vi "Methods to Method Info.vi"(10 "Class":string, 11 "Methods from Node":T2(array[cluster])) -> (2 "Methods for Tree":T1(array[cluster]), 3 "Methods[]":T3(array[cluster])=[{"Class Info"={"Unique ID string"="1", "Parent ID string"="", "Class Name (unlocalized)"="Application", "Class Name (localized)"="Application"}, "Method Info"={"Unique ID string"="7d0", "Data name"="Print.Function To Printer", "Short name (localized)"="Print.Function To Printer", "Long name (localized)"="Print:Function To Printer"}, "Method Flags"={"IsDeprecated"=FALSE, "IsPrivate"=TRUE, "IsScripting"=FALSE, "IsNotInRun-Time"=TRUE}, "Divider"=FALSE}, {"Class Info"={"Unique ID string"="1", "Parent ID string"="", "Class Name (unlocalized)"="Application", "Class Name (localized)"="Application"}, "Method Info"={"Unique ID string"="7d5", "Data name"="Mass Compile", "Short name (localized)"="Mass Compile", "Long name (localized)"="Mass Compile"}, "Method Flags"={"IsDeprecated"=FALSE, "IsPrivate"=FALSE, "IsScripting"=FALSE, "IsNotInRun-Time"=TRUE}, "Divider"=FALSE}, {"Class Info"={"Unique ID string"="1", "Parent ID string"="", "Class Name (unlocalized)"="Application", "Class Name (localized)"="Application"}, "Method Info"={"Unique ID string"="7d6", "Data name"="UI.Cmp VIs", "Short name (localized)"="UI.Cmp VIs", "Long name (localized)"="User Interaction:Compare VIs"}, "Method Flags"={"IsDeprecated"=FALSE, "IsPrivate"=TRUE, "IsScripting"=FALSE, "IsNotInRun-Time"=TRUE}, "Divider"=FALSE}, {"Class Info"={"Unique ID string"="1", "Parent ID string"="", "Class Name (unlocalized)"="Application", "Class Name (localized)"="Application"}, "Method Info"={"Unique ID string"="7da", "Data name"="History Since", "Short name (localized)"="History Since", "Long name (localized)"="History Since"}, "Method Flags"={"IsDeprecated"=FALSE, "IsPrivate"=TRUE, "IsScripting"=FALSE, "IsNotInRun-Time"=TRUE}, "Divider"=FALSE}, {"Class Info"={"Unique ID string"="1", "Parent ID string"="", "Class Name (unlocalized)"="Application", "Class Name (localized)"="Application"}, "Method Info"={"Unique ID string"="7de", "Data name"="Bring To Front", "Short name (localized)"="Bring To Front", "Long name (localized)"="Bring To Front"}, "Method Flags"={"IsDeprecated"=FALSE, "IsPrivate"=FALSE, "IsScripting"=FALSE, "IsNotInRun-Time"=FALSE}, "Divider"=FALSE}, {"Class Info"={"Unique ID string"="1", "Parent ID string"="", "Class Name (unlocalized)"="Application", "Class Name (localized)"="Application"}, "Method Info"={"Unique ID string"="7e0", "Data name"="Build.Application", "Short name (localized)"="Build.Application", "Long name (localized)"="Build:Application"}, "Method Flags"={"IsDeprecated"=FALSE, "IsPrivate"=TRUE, "IsScripting"=FALSE, "IsNotInRun-Time"=TRUE}, "Divider"=FALSE}, {"Class Info"={"Unique ID string"="1", "Parent ID string"="", "Class Name (unlocalized)"="Application", "Class Name (localized)"="Application"}, "Method Info"={"Unique ID string"="7e1", "Data name"="Build.Distribution", "Short name (localized)"="Build.Distribution", "Long name (localized)"="Build:Distribution"}, "Method Flags"={"IsDeprecated"=FALSE, "IsPrivate"=TRUE, "IsScripting"=FALSE, "IsNotInRun-Time"=TRUE}, "Divider"=FALSE}, {"Class Info"={"Unique ID string"="1", "Parent ID string"="", "Class Name (unlocalized)"="Application", "Class Name (localized)"="Application"}, "Method Info"={"Unique ID string"="7e3", "Data name"="Disconnect From Slave", "Short name (localized)"="Disconnect From Slave", "Long name (localized)"="LVRT:Disconnect From Slave"}, "Method Flags"={"IsDeprecated"=FALSE, "IsPrivate"=FALSE, "IsScripting"=FALSE, "IsNotInRun-Time"=TRUE}, "Divider"=FALSE}, {"Class Info"={"Unique ID string"="1", "Parent ID string"="", "Class Name (unlocalized)"="Application", "Class Name (localized)"="Application"}, "Method Info"={"Unique ID string"="7e4", "Data name"="LVRT.Check DLLs", "Short name (localized)"="LVRT.Check DLLs", "Long name (localized)"="LVRT:Check DLLs"}, "Method Flags"={"IsDeprecated"=FALSE, "IsPrivate"=TRUE, "IsScripting"=FALSE, "IsNotInRun-Time"=TRUE}, "Divider"=FALSE}, {"Class Info"={"Unique ID string"="1", "Parent ID string"="", "Class Name (unlocalized)"="Application", "Class Name (localized)"="Application"}, "Method Info"={"Unique ID string"="7e6", "Data name"="Call Internal Cmd", "Short name (localized)"="Call Internal Cmd", "Long name (localized)"="Call Internal Command"}, "Method Flags"={"IsDeprecated"=FALSE, "IsPrivate"=TRUE, "IsScripting"=FALSE, "IsNotInRun-Time"=FALSE}, "Divider"=FALSE}, {"Class Info"={"Unique ID string"="1", "Parent ID string"="", "Class Name (unlocalized)"="Application", "Class Name (localized)"="Application"}, "Method Info"={"Unique ID string"="7e7", "Data name"="Query Internal Operation Tracking Data", "Short name (localized)"="Query Internal Operation Tracking Data", "Long name (localized)"="Query Internal Operation Tracking Data"}, "Method Flags"={"IsDeprecated"=FALSE, "IsPrivate"=TRUE, "IsScripting"=FALSE, "IsNotInRun-Time"=FALSE}, "Divider"=FALSE}, {"Class Info"={"Unique ID string"="1", "Parent ID string"="", "Class Name (unlocalized)"="Application", "Class Name (localized)"="Application"}, "Method Info"={"Unique ID string"="7e8", "Data name"="Class Operator.Get", "Short name (localized)"="Class Operator.Get", "Long name (localized)"="Class Operator:Get"}, "Method Flags"={"IsDeprecated"=FALSE, "IsPrivate"=FALSE, "IsScripting"=TRUE, "IsNotInRun-Time"=FALSE}, "Divider"=FALSE}, {"Class Info"={"Unique ID string"="1", "Parent ID string"="", "Class Name (unlocalized)"="Application", "Class Name (localized)"="Application"}, "Method Info"={"Unique ID string"="7e9", "Data name"="Class Operator.Set", "Short name (localized)"="Class Operator.Set", "Long name (localized)"="Class Operator:Set"}, "Method Flags"={"IsDeprecated"=FALSE, "IsPrivate"=FALSE, "IsScripting"=TRUE, "IsNotInRun-Time"=FALSE}, "Divider"=FALSE}, {"Class Info"={"Unique ID string"="1", "Parent ID string"="", "Class Name (unlocalized)"="Application", "Class Name (localized)"="Application"}, "Method Info"={"Unique ID string"="7ea", "Data name"="Class Operator.Remove", "Short name (localized)"="Class Operator.Remove", "Long name (localized)"="Class Operator:Remove"}, "Method Flags"={"IsDeprecated"=FALSE, "IsPrivate"=FALSE, "IsScripting"=TRUE, "IsNotInRun-Time"=FALSE}, "Divider"=FALSE}, {"Class Info"={"Unique ID string"="1", "Parent ID string"="", "Class Name (unlocalized)"="Application", "Class Name (localized)"="Application"}, "Method Info"={"Unique ID string"="7eb", "Data name"="Class Operator.Remove All", "Short name (localized)"="Class Operator.Remove All", "Long name (localized)"="Class Operator:Remove All"}, "Method Flags"={"IsDeprecated"=FALSE, "IsPrivate"=FALSE, "IsScripting"=TRUE, "IsNotInRun-Time"=FALSE}, "Divider"=FALSE}, {"Class Info"={"Unique ID string"="1", "Parent ID string"="", "Class Name (unlocalized)"="Application", "Class Name (localized)"="Application"}, "Method Info"={"Unique ID string"="7ed", "Data name"="Clipboard.Get Image", "Short name (localized)"="Clipboard.Get Image", "Long name (localized)"="Clipboard:Get Image"}, "Method Flags"={"IsDeprecated"=FALSE, "IsPrivate"=FALSE, "IsScripting"=FALSE, "IsNotInRun-Time"=FALSE}, "Divider"=FALSE}, {"Class Info"={"Unique ID string"="1", "Parent ID string"="", "Class Name (unlocalized)"="Application", "Class Name (localized)"="Application"}, "Method Info"={"Unique ID string"="7ee", "Data name"="RP.Server Network Load", "Short name (localized)"="RP.Server Network Load", "Long name (localized)"="Remote Panel:Server Network Load"}, "Method Flags"={"IsDeprecated"=FALSE, "IsPrivate"=TRUE, "IsScripting"=FALSE, "IsNotInRun-Time"=FALSE}, "Divider"=FALSE}, {"Class Info"={"Unique ID string"="1", "Parent ID string"="", "Class Name (unlocalized)"="Application", "Class Name (localized)"="Application"}, "Method Info"={"Unique ID string"="7ef", "Data name"="Clipboard.Empty", "Short name (localized)"="Clipboard.Empty", "Long name (localized)"="Clipboard:Empty"}, "Method Flags"={"IsDeprecated"=FALSE, "IsPrivate"=FALSE, "IsScripting"=TRUE, "IsNotInRun-Time"=TRUE}, "Divider"=FALSE}, {"Class Info"={"Unique ID string"="1", "Parent ID string"="", "Class Name (unlocalized)"="Application", "Class Name (localized)"="Application"}, "Method Info"={"Unique ID string"="7f1", "Data name"="RP.Open Connection To Server", "Short name (localized)"="RP.Open Connection To Server", "Long name (localized)"="Remote Panel:Open Connection To Server"}, "Method Flags"={"IsDeprecated"=FALSE, "IsPrivate"=FALSE, "IsScripting"=FALSE, "IsNotInRun-Time"=FALSE}, "Divider"=FALSE}, {"Class Info"={"Unique ID string"="1", "Parent ID string"="", "Class Name (unlocalized)"="Application", "Class Name (localized)"="Application"}, "Method Info"={"Unique ID string"="7f2", "Data name"="RP.Client Network Load", "Short name (localized)"="RP.Client Network Load", "Long name (localized)"="Remote Panel:Client Network Load"}, "Method Flags"={"IsDeprecated"=FALSE, "IsPrivate"=TRUE, "IsScripting"=FALSE, "IsNotInRun-Time"=FALSE}, "Divider"=FALSE}, {"Class Info"={"Unique ID string"="1", "Parent ID string"="", "Class Name (unlocalized)"="Application", "Class Name (localized)"="Application"}, "Method Info"={"Unique ID string"="7f3", "Data name"="Compile VIs Needing Compilation", "Short name (localized)"="Compile VIs Needing Compilation", "Long name (localized)"="Compile VIs Needing Compilation"}, "Method Flags"={"IsDeprecated"=FALSE, "IsPrivate"=TRUE, "IsScripting"=FALSE, "IsNotInRun-Time"=TRUE}, "Divider"=FALSE}, {"Class Info"={"Unique ID string"="1", "Parent ID string"="", "Class Name (unlocalized)"="Application", "Class Name (localized)"="Application"}, "Method Info"={"Unique ID string"="7f4", "Data name"="UI.Show Inplaceness Terminals", "Short name (localized)"="UI.Show Inplaceness Terminals", "Long name (localized)"="User Interaction:Show Inplaceness Terminals"}, "Method Flags"={"IsDeprecated"=FALSE, "IsPrivate"=TRUE, "IsScripting"=FALSE, "IsNotInRun-Time"=TRUE}, "Divider"=FALSE}, {"Class Info"={"Unique ID string"="1", "Parent ID string"="", "Class Name (unlocalized)"="Application", "Class Name (localized)"="Application"}, "Method Info"={"Unique ID string"="7f7", "Data name"="Conn Responsive.Check", "Short name (localized)"="Conn Responsive.Check", "Long name (localized)"="Connection Responsiveness:Check"}, "Method Flags"={"IsDeprecated"=FALSE, "IsPrivate"=FALSE, "IsScripting"=FALSE, "IsNotInRun-Time"=FALSE}, "Divider"=FALSE}, {"Class Info"={"Unique ID string"="1", "Parent ID string"="", "Class Name (unlocalized)"="Application", "Class Name (localized)"="Application"}, "Method Info"={"Unique ID string"="7f8", "Data name"="Conn Responsive.Info", "Short name (localized)"="Conn Responsive.Info", "Long name (localized)"="Connection Responsiveness:Information"}, "Method Flags"={"IsDeprecated"=FALSE, "IsPrivate"=FALSE, "IsScripting"=FALSE, "IsNotInRun-Time"=FALSE}, "Divider"=FALSE}, {"Class Info"={"Unique ID string"="1", "Parent ID string"="", "Class Name (unlocalized)"="Application", "Class Name (localized)"="Application"}, "Method Info"={"Unique ID string"="7f9", "Data name"="Get VI Version", "Short name (localized)"="Get VI Version", "Long name (localized)"="Get VI:Version"}, "Method Flags"={"IsDeprecated"=FALSE, "IsPrivate"=FALSE, "IsScripting"=FALSE, "IsNotInRun-Time"=FALSE}, "Divider"=FALSE}, {"Class Info"={"Unique ID string"="1", "Parent ID string"="", "Class Name (unlocalized)"="Application", "Class Name (localized)"="Application"}, "Method Info"={"Unique ID string"="7fa", "Data name"="UI.PlacePaletteObjOnCursor", "Short name (localized)"="UI.PlacePaletteObjOnCursor", "Long name (localized)"="User Interaction:Place Palette Object on Cursor"}, "Method Flags"={"IsDeprecated"=FALSE, "IsPrivate"=FALSE, "IsScripting"=TRUE, "IsNotInRun-Time"=TRUE}, "Divider"=FALSE}, {"Class Info"={"Unique ID string"="1", "Parent ID string"="", "Class Name (unlocalized)"="Application", "Class Name (localized)"="Application"}, "Method Info"={"Unique ID string"="7fb", "Data name"="Browse DataSocket", "Short name (localized)"="Browse DataSocket", "Long name (localized)"="Browse DataSocket"}, "Method Flags"={"IsDeprecated"=FALSE, "IsPrivate"=FALSE, "IsScripting"=FALSE, "IsNotInRun-Time"=FALSE}, "Divider"=FALSE}, {"Class Info"={"Unique ID string"="1", "Parent ID string"="", "Class Name (unlocalized)"="Application", "Class Name (localized)"="Application"}, "Method Info"={"Unique ID string"="7fd", "Data name"="UI.Hilight Pal Menu Item", "Short name (localized)"="UI.Hilight Pal Menu Item", "Long name (localized)"="User Interaction:Hilight Palette Menu Item"}, "Method Flags"={"IsDeprecated"=FALSE, "IsPrivate"=FALSE, "IsScripting"=TRUE, "IsNotInRun-Time"=TRUE}, "Divider"=FALSE}, {"Class Info"={"Unique ID string"="1", "Parent ID string"="", "Class Name (unlocalized)"="Application", "Class Name (localized)"="Application"}, "Method Info"={"Unique ID string"="7ff", "Data name"="New LabVIEW Document", "Short name (localized)"="New LabVIEW Document", "Long name (localized)"="New LabVIEW Document"}, "Method Flags"={"IsDeprecated"=FALSE, "IsPrivate"=FALSE, "IsScripting"=TRUE, "IsNotInRun-Time"=TRUE}, "Divider"=FALSE}, {"Class Info"={"Unique ID string"="1", "Parent ID string"="", "Class Name (unlocalized)"="Application", "Class Name (localized)"="Application"}, "Method Info"={"Unique ID string"="800", "Data name"="Pwd.Clear Cache", "Short name (localized)"="Pwd.Clear Cache", "Long name (localized)"="Password:Clear Cache"}, "Method Flags"={"IsDeprecated"=FALSE, "IsPrivate"=TRUE, "IsScripting"=FALSE, "IsNotInRun-Time"=FALSE}, "Divider"=FALSE}, {"Class Info"={"Unique ID string"="1", "Parent ID string"="", "Class Name (unlocalized)"="Application", "Class Name (localized)"="Application"}, "Method Info"={"Unique ID string"="801", "Data name"="Pwd.Add To Cache", "Short name (localized)"="Pwd.Add To Cache", "Long name (localized)"="Password:Add To Cache"}, "Method Flags"={"IsDeprecated"=FALSE, "IsPrivate"=TRUE, "IsScripting"=FALSE, "IsNotInRun-Time"=FALSE}, "Divider"=FALSE}, {"Class Info"={"Unique ID string"="1", "Parent ID string"="", "Class Name (unlocalized)"="Application", "Class Name (localized)"="Application"}, "Method Info"={"Unique ID string"="802", "Data name"="RP.Close Connection To Server", "Short name (localized)"="RP.Close Connection To Server", "Long name (localized)"="Remote Panel:Close Connection To Server"}, "Method Flags"={"IsDeprecated"=FALSE, "IsPrivate"=FALSE, "IsScripting"=FALSE, "IsNotInRun-Time"=FALSE}, "Divider"=FALSE}, {"Class Info"={"Unique ID string"="1", "Parent ID string"="", "Class Name (unlocalized)"="Application", "Class Name (localized)"="Application"}, "Method Info"={"Unique ID string"="803", "Data name"="RP.Client Request Control", "Short name (localized)"="RP.Client Request Control", "Long name (localized)"="Remote Panel:Client Request Control"}, "Method Flags"={"IsDeprecated"=FALSE, "IsPrivate"=FALSE, "IsScripting"=FALSE, "IsNotInRun-Time"=FALSE}, "Divider"=FALSE}, {"Class Info"={"Unique ID string"="1", "Parent ID string"="", "Class Name (unlocalized)"="Application", "Class Name (localized)"="Application"}, "Method Info"={"Unique ID string"="804", "Data name"="RP.Client Release Control", "Short name (localized)"="RP.Client Release Control", "Long name (localized)"="Remote Panel:Client Release Control"}, "Method Flags"={"IsDeprecated"=FALSE, "IsPrivate"=FALSE, "IsScripting"=FALSE, "IsNotInRun-Time"=FALSE}, "Divider"=FALSE}, {"Class Info"={"Unique ID string"="1", "Parent ID string"="", "Class Name (unlocalized)"="Application", "Class Name (localized)"="Application"}, "Method Info"={"Unique ID string"="805", "Data name"="Get VI.Title", "Short name (localized)"="Get VI.Title", "Long name (localized)"="Get VI:Title"}, "Method Flags"={"IsDeprecated"=FALSE, "IsPrivate"=FALSE, "IsScripting"=FALSE, "IsNotInRun-Time"=FALSE}, "Divider"=FALSE}, {"Class Info"={"Unique ID string"="1", "Parent ID string"="", "Class Name (unlocalized)"="Application", "Class Name (localized)"="Application"}, "Method Info"={"Unique ID string"="806", "Data name"="Get VI.Description", "Short name (localized)"="Get VI.Description", "Long name (localized)"="Get VI:Description"}, "Method Flags"={"IsDeprecated"=FALSE, "IsPrivate"=FALSE, "IsScripting"=FALSE, "IsNotInRun-Time"=FALSE}, "Divider"=FALSE}, {"Class Info"={"Unique ID string"="1", "Parent ID string"="", "Class Name (unlocalized)"="Application", "Class Name (localized)"="Application"}, "Method Info"={"Unique ID string"="807", "Data name"="Add Probe To Cache", "Short name (localized)"="Add Probe To Cache", "Long name (localized)"="Add Probe To Cache"}, "Method Flags"={"IsDeprecated"=FALSE, "IsPrivate"=TRUE, "IsScripting"=FALSE, "IsNotInRun-Time"=FALSE}, "Divider"=FALSE}, {"Class Info"={"Unique ID string"="1", "Parent ID string"="", "Class Name (unlocalized)"="Application", "Class Name (localized)"="Application"}, "Method Info"={"Unique ID string"="809", "Data name"="Create COM WDT Data", "Short name (localized)"="Create COM WDT Data", "Long name (localized)"="Create COM WDT Data"}, "Method Flags"={"IsDeprecated"=FALSE, "IsPrivate"=TRUE, "IsScripting"=FALSE, "IsNotInRun-Time"=FALSE}, "Divider"=FALSE}, {"Class Info"={"Unique ID string"="1", "Parent ID string"="", "Class Name (unlocalized)"="Application", "Class Name (localized)"="Application"}, "Method Info"={"Unique ID string"="80a", "Data name"="Image Data To Byte Array", "Short name (localized)"="Image Data To Byte Array", "Long name (localized)"="Image Data To Byte Array"}, "Method Flags"={"IsDeprecated"=FALSE, "IsPrivate"=TRUE, "IsScripting"=FALSE, "IsNotInRun-Time"=FALSE}, "Divider"=FALSE}, {"Class Info"={"Unique ID string"="1", "Parent ID string"="", "Class Name (unlocalized)"="Application", "Class Name (localized)"="Application"}, "Method Info"={"Unique ID string"="80b", "Data name"=".NET.Get Assembly Full Name", "Short name (localized)"=".NET.Get Assembly Full Name", "Long name (localized)"=".NET:Get Assembly Full Name"}, "Method Flags"={"IsDeprecated"=FALSE, "IsPrivate"=TRUE, "IsScripting"=FALSE, "IsNotInRun-Time"=TRUE}, "Divider"=FALSE}, {"Class Info"={"Unique ID string"="1", "Parent ID string"="", "Class Name (unlocalized)"="Application", "Class Name (localized)"="Application"}, "Method Info"={"Unique ID string"="80c", "Data name"=".NET.Convert To .NET Type", "Short name (localized)"=".NET.Convert To .NET Type", "Long name (localized)"=".NET:Convert To .NET Type"}, "Method Flags"={"IsDeprecated"=FALSE, "IsPrivate"=TRUE, "IsScripting"=FALSE, "IsNotInRun-Time"=FALSE}, "Divider"=FALSE}, {"Class Info"={"Unique ID string"="1", "Parent ID string"="", "Class Name (unlocalized)"="Application", "Class Name (localized)"="Application"}, "Method Info"={"Unique ID string"="80d", "Data name"=".NET.Convert Obj To LV Variant", "Short name (localized)"=".NET.Convert Obj To LV Variant", "Long name (localized)"=".NET:Convert Object To LabVIEW Variant"}, "Method Flags"={"IsDeprecated"=FALSE, "IsPrivate"=TRUE, "IsScripting"=FALSE, "IsNotInRun-Time"=FALSE}, "Divider"=FALSE}, {"Class Info"={"Unique ID string"="1", "Parent ID string"="", "Class Name (unlocalized)"="Application", "Class Name (localized)"="Application"}, "Method Info"={"Unique ID string"="80e", "Data name"="Get Pal Menu Info", "Short name (localized)"="Get Pal Menu Info", "Long name (localized)"="Palettes:Get Menu Information"}, "Method Flags"={"IsDeprecated"=FALSE, "IsPrivate"=TRUE, "IsScripting"=FALSE, "IsNotInRun-Time"=TRUE}, "Divider"=FALSE}, {"Class Info"={"Unique ID string"="1", "Parent ID string"="", "Class Name (unlocalized)"="Application", "Class Name (localized)"="Application"}, "Method Info"={"Unique ID string"="810", "Data name"="C TypeDefs.Reset", "Short name (localized)"="C TypeDefs.Reset", "Long name (localized)"="C TypeDefs:Reset"}, "Method Flags"={"IsDeprecated"=FALSE, "IsPrivate"=TRUE, "IsScripting"=FALSE, "IsNotInRun-Time"=FALSE}, "Divider"=FALSE}, {"Class Info"={"Unique ID string"="1", "Parent ID string"="", "Class Name (unlocalized)"="Application", "Class Name (localized)"="Application"}, "Method Info"={"Unique ID string"="811", "Data name"="C TypeDefs.Get", "Short name (localized)"="C TypeDefs.Get", "Long name (localized)"="C TypeDefs:Get"}, "Method Flags"={"IsDeprecated"=FALSE, "IsPrivate"=TRUE, "IsScripting"=FALSE, "IsNotInRun-Time"=FALSE}, "Divider"=FALSE}, {"Class Info"={"Unique ID string"="1", "Parent ID string"="", "Class Name (unlocalized)"="Application", "Class Name (localized)"="Application"}, "Method Info"={"Unique ID string"="812", "Data name"="Context.OpenSibling", "Short name (localized)"="Context.OpenSibling", "Long name (localized)"="Context:Open Sibling"}, "Method Flags"={"IsDeprecated"=FALSE, "IsPrivate"=TRUE, "IsScripting"=FALSE, "IsNotInRun-Time"=FALSE}, "Divider"=FALSE}, {"Class Info"={"Unique ID string"="1", "Parent ID string"="", "Class Name (unlocalized)"="Application", "Class Name (localized)"="Application"}, "Method Info"={"Unique ID string"="813", "Data name"="Project.Open", "Short name (localized)"="Project.Open", "Long name (localized)"="Project:Open"}, "Method Flags"={"IsDeprecated"=FALSE, "IsPrivate"=FALSE, "IsScripting"=FALSE, "IsNotInRun-Time"=FALSE}, "Divider"=FALSE}, {"Class Info"={"Unique ID string"="1", "Parent ID string"="", "Class Name (unlocalized)"="Application", "Class Name (localized)"="Application"}, "Method Info"={"Unique ID string"="814", "Data name"="Project.New", "Short name (localized)"="Project.New", "Long name (localized)"="Project:New"}, "Method Flags"={"IsDeprecated"=FALSE, "IsPrivate"=FALSE, "IsScripting"=FALSE, "IsNotInRun-Time"=TRUE}, "Divider"=FALSE}, {"Class Info"={"Unique ID string"="1", "Parent ID string"="", "Class Name (unlocalized)"="Application", "Class Name (localized)"="Application"}, "Method Info"={"Unique ID string"="815", "Data name"="Context.CreateLocalHostAppInstance", "Short name (localized)"="Context.CreateLocalHostAppInstance", "Long name (localized)"="Context:Create Local Host App Instance"}, "Method Flags"={"IsDeprecated"=FALSE, "IsPrivate"=TRUE, "IsScripting"=FALSE, "IsNotInRun-Time"=FALSE}, "Divider"=FALSE}, {"Class Info"={"Unique ID string"="1", "Parent ID string"="", "Class Name (unlocalized)"="Application", "Class Name (localized)"="Application"}, "Method Info"={"Unique ID string"="816", "Data name"="Linker.Notify of File Change", "Short name (localized)"="Linker.Notify of File Change", "Long name (localized)"="Linker:Notify of File Change"}, "Method Flags"={"IsDeprecated"=FALSE, "IsPrivate"=TRUE, "IsScripting"=TRUE, "IsNotInRun-Time"=TRUE}, "Divider"=FALSE}, {"Class Info"={"Unique ID string"="1", "Parent ID string"="", "Class Name (unlocalized)"="Application", "Class Name (localized)"="Application"}, "Method Info"={"Unique ID string"="817", "Data name"="Project.Get New Items", "Short name (localized)"="Project.Get New Items", "Long name (localized)"="Project:Get New Items"}, "Method Flags"={"IsDeprecated"=FALSE, "IsPrivate"=TRUE, "IsScripting"=FALSE, "IsNotInRun-Time"=FALSE}, "Divider"=FALSE}, {"Class Info"={"Unique ID string"="1", "Parent ID string"="", "Class Name (unlocalized)"="Application", "Class Name (localized)"="Application"}, "Method Info"={"Unique ID string"="818", "Data name"="Project.Do New Item", "Short name (localized)"="Project.Do New Item", "Long name (localized)"="Project:Do New Item"}, "Method Flags"={"IsDeprecated"=FALSE, "IsPrivate"=TRUE, "IsScripting"=FALSE, "IsNotInRun-Time"=TRUE}, "Divider"=FALSE}, {"Class Info"={"Unique ID string"="1", "Parent ID string"="", "Class Name (unlocalized)"="Application", "Class Name (localized)"="Application"}, "Method Info"={"Unique ID string"="81a", "Data name"="UI.Invoke Menu Item", "Short name (localized)"="UI.Invoke Menu Item", "Long name (localized)"="User Interaction:Invoke Menu Item"}, "Method Flags"={"IsDeprecated"=FALSE, "IsPrivate"=FALSE, "IsScripting"=TRUE, "IsNotInRun-Time"=FALSE}, "Divider"=FALSE}, {"Class Info"={"Unique ID string"="1", "Parent ID string"="", "Class Name (unlocalized)"="Application", "Class Name (localized)"="Application"}, "Method Info"={"Unique ID string"="81b", "Data name"="Open.LV Document", "Short name (localized)"="Open.LV Document", "Long name (localized)"="Open:LabVIEW Document"}, "Method Flags"={"IsDeprecated"=FALSE, "IsPrivate"=FALSE, "IsScripting"=TRUE, "IsNotInRun-Time"=TRUE}, "Divider"=FALSE}, {"Class Info"={"Unique ID string"="1", "Parent ID string"="", "Class Name (unlocalized)"="Application", "Class Name (localized)"="Application"}, "Method Info"={"Unique ID string"="81c", "Data name"="RecentOpen.LV Files", "Short name (localized)"="RecentOpen.LV Files", "Long name (localized)"="Recently Opened:LV Files"}, "Method Flags"={"IsDeprecated"=FALSE, "IsPrivate"=FALSE, "IsScripting"=TRUE, "IsNotInRun-Time"=TRUE}, "Divider"=FALSE}, {"Class Info"={"Unique ID string"="1", "Parent ID string"="", "Class Name (unlocalized)"="Application", "Class Name (localized)"="Application"}, "Method Info"={"Unique ID string"="81d", "Data name"="UI.Search LabVIEW Help", "Short name (localized)"="UI.Search LabVIEW Help", "Long name (localized)"="User Interaction:Search LabVIEW Help"}, "Method Flags"={"IsDeprecated"=FALSE, "IsPrivate"=TRUE, "IsScripting"=FALSE, "IsNotInRun-Time"=TRUE}, "Divider"=FALSE}, {"Class Info"={"Unique ID string"="1", "Parent ID string"="", "Class Name (unlocalized)"="Application", "Class Name (localized)"="Application"}, "Method Info"={"Unique ID string"="81e", "Data name"="Context.Get Preferred", "Short name (localized)"="Context.Get Preferred", "Long name (localized)"="Context:Get Preferred"}, "Method Flags"={"IsDeprecated"=FALSE, "IsPrivate"=TRUE, "IsScripting"=FALSE, "IsNotInRun-Time"=FALSE}, "Divider"=FALSE}, {"Class Info"={"Unique ID string"="1", "Parent ID string"="", "Class Name (unlocalized)"="Application", "Class Name (localized)"="Application"}, "Method Info"={"Unique ID string"="81f", "Data name"="License.Check Out", "Short name (localized)"="License.Check Out", "Long name (localized)"="License:Check Out"}, "Method Flags"={"IsDeprecated"=FALSE, "IsPrivate"=TRUE, "IsScripting"=FALSE, "IsNotInRun-Time"=FALSE}, "Divider"=FALSE}, {"Class Info"={"Unique ID string"="1", "Parent ID string"="", "Class Name (unlocalized)"="Application", "Class Name (localized)"="Application"}, "Method Info"={"Unique ID string"="820", "Data name"="License.Check In", "Short name (localized)"="License.Check In", "Long name (localized)"="License:Check In"}, "Method Flags"={"IsDeprecated"=FALSE, "IsPrivate"=TRUE, "IsScripting"=FALSE, "IsNotInRun-Time"=FALSE}, "Divider"=FALSE}, {"Class Info"={"Unique ID string"="1", "Parent ID string"="", "Class Name (unlocalized)"="Application", "Class Name (localized)"="Application"}, "Method Info"={"Unique ID string"="823", "Data name"="Config.Get Settings", "Short name (localized)"="Config.Get Settings", "Long name (localized)"="Configuration:Get Settings"}, "Method Flags"={"IsDeprecated"=FALSE, "IsPrivate"=TRUE, "IsScripting"=FALSE, "IsNotInRun-Time"=FALSE}, "Divider"=FALSE}, {"Class Info"={"Unique ID string"="1", "Parent ID string"="", "Class Name (unlocalized)"="Application", "Class Name (localized)"="Application"}, "Method Info"={"Unique ID string"="825", "Data name"="Library.Open", "Short name (localized)"="Library.Open", "Long name (localized)"="Library:Open"}, "Method Flags"={"IsDeprecated"=FALSE, "IsPrivate"=FALSE, "IsScripting"=FALSE, "IsNotInRun-Time"=FALSE}, "Divider"=FALSE}, {"Class Info"={"Unique ID string"="1", "Parent ID string"="", "Class Name (unlocalized)"="Application", "Class Name (localized)"="Application"}, "Method Info"={"Unique ID string"="826", "Data name"="Library.Create", "Short name (localized)"="Library.Create", "Long name (localized)"="Library:Create"}, "Method Flags"={"IsDeprecated"=FALSE, "IsPrivate"=FALSE, "IsScripting"=FALSE, "IsNotInRun-Time"=TRUE}, "Divider"=FALSE}, {"Class Info"={"Unique ID string"="1", "Parent ID string"="", "Class Name (unlocalized)"="Application", "Class Name (localized)"="Application"}, "Method Info"={"Unique ID string"="827", "Data name"="NI Security.Login", "Short name (localized)"="NI Security.Login", "Long name (localized)"="NI Security:Login"}, "Method Flags"={"IsDeprecated"=FALSE, "IsPrivate"=FALSE, "IsScripting"=FALSE, "IsNotInRun-Time"=FALSE}, "Divider"=FALSE}, {"Class Info"={"Unique ID string"="1", "Parent ID string"="", "Class Name (unlocalized)"="Application", "Class Name (localized)"="Application"}, "Method Info"={"Unique ID string"="828", "Data name"="NI Security.Logout", "Short name (localized)"="NI Security.Logout", "Long name (localized)"="NI Security:Logout"}, "Method Flags"={"IsDeprecated"=FALSE, "IsPrivate"=FALSE, "IsScripting"=FALSE, "IsNotInRun-Time"=FALSE}, "Divider"=FALSE}, {"Class Info"={"Unique ID string"="1", "Parent ID string"="", "Class Name (unlocalized)"="Application", "Class Name (localized)"="Application"}, "Method Info"={"Unique ID string"="829", "Data name"="NI Security.Invoke Login Dialog", "Short name (localized)"="NI Security.Invoke Login Dialog", "Long name (localized)"="NI Security:Invoke Login Dialog"}, "Method Flags"={"IsDeprecated"=FALSE, "IsPrivate"=FALSE, "IsScripting"=FALSE, "IsNotInRun-Time"=FALSE}, "Divider"=FALSE}, {"Class Info"={"Unique ID string"="1", "Parent ID string"="", "Class Name (unlocalized)"="Application", "Class Name (localized)"="Application"}, "Method Info"={"Unique ID string"="82a", "Data name"="NI Security.Get Access Rights", "Short name (localized)"="NI Security.Get Access Rights", "Long name (localized)"="NI Security:Get Access Rights"}, "Method Flags"={"IsDeprecated"=FALSE, "IsPrivate"=FALSE, "IsScripting"=FALSE, "IsNotInRun-Time"=FALSE}, "Divider"=FALSE}, {"Class Info"={"Unique ID string"="1", "Parent ID string"="", "Class Name (unlocalized)"="Application", "Class Name (localized)"="Application"}, "Method Info"={"Unique ID string"="82b", "Data name"="I/O Ctrl.Get Names", "Short name (localized)"="I/O Ctrl.Get Names", "Long name (localized)"="I/O Control:Get Names"}, "Method Flags"={"IsDeprecated"=FALSE, "IsPrivate"=TRUE, "IsScripting"=FALSE, "IsNotInRun-Time"=FALSE}, "Divider"=FALSE}, {"Class Info"={"Unique ID string"="1", "Parent ID string"="", "Class Name (unlocalized)"="Application", "Class Name (localized)"="Application"}, "Method Info"={"Unique ID string"="82c", "Data name"="I/O Ctrl.Get Name Attributes", "Short name (localized)"="I/O Ctrl.Get Name Attributes", "Long name (localized)"="I/O Control:Get Name Attributes"}, "Method Flags"={"IsDeprecated"=FALSE, "IsPrivate"=TRUE, "IsScripting"=FALSE, "IsNotInRun-Time"=FALSE}, "Divider"=FALSE}, {"Class Info"={"Unique ID string"="1", "Parent ID string"="", "Class Name (unlocalized)"="Application", "Class Name (localized)"="Application"}, "Method Info"={"Unique ID string"="82f", "Data name"="Project.Reg Proj Ref For Cleanup Proc", "Short name (localized)"="Project.Reg Proj Ref For Cleanup Proc", "Long name (localized)"="Project:Register Proj Ref For Cleanup Proc"}, "Method Flags"={"IsDeprecated"=FALSE, "IsPrivate"=TRUE, "IsScripting"=FALSE, "IsNotInRun-Time"=TRUE}, "Divider"=FALSE}, {"Class Info"={"Unique ID string"="1", "Parent ID string"="", "Class Name (unlocalized)"="Application", "Class Name (localized)"="Application"}, "Method Info"={"Unique ID string"="830", "Data name"="Open.Recently Opened File", "Short name (localized)"="Open.Recently Opened File", "Long name (localized)"="Open:Recently Opened File"}, "Method Flags"={"IsDeprecated"=FALSE, "IsPrivate"=FALSE, "IsScripting"=TRUE, "IsNotInRun-Time"=FALSE}, "Divider"=FALSE}, {"Class Info"={"Unique ID string"="1", "Parent ID string"="", "Class Name (unlocalized)"="Application", "Class Name (localized)"="Application"}, "Method Info"={"Unique ID string"="831", "Data name"="XControl.Create", "Short name (localized)"="XControl.Create", "Long name (localized)"="XControl:Create"}, "Method Flags"={"IsDeprecated"=FALSE, "IsPrivate"=FALSE, "IsScripting"=FALSE, "IsNotInRun-Time"=TRUE}, "Divider"=FALSE}, {"Class Info"={"Unique ID string"="1", "Parent ID string"="", "Class Name (unlocalized)"="Application", "Class Name (localized)"="Application"}, "Method Info"={"Unique ID string"="832", "Data name"="XNode.Create", "Short name (localized)"="XNode.Create", "Long name (localized)"="XNode:Create"}, "Method Flags"={"IsDeprecated"=FALSE, "IsPrivate"=TRUE, "IsScripting"=FALSE, "IsNotInRun-Time"=TRUE}, "Divider"=FALSE}, {"Class Info"={"Unique ID string"="1", "Parent ID string"="", "Class Name (unlocalized)"="Application", "Class Name (localized)"="Application"}, "Method Info"={"Unique ID string"="833", "Data name"="XControl.Open", "Short name (localized)"="XControl.Open", "Long name (localized)"="XControl:Open"}, "Method Flags"={"IsDeprecated"=FALSE, "IsPrivate"=FALSE, "IsScripting"=FALSE, "IsNotInRun-Time"=TRUE}, "Divider"=FALSE}, {"Class Info"={"Unique ID string"="1", "Parent ID string"="", "Class Name (unlocalized)"="Application", "Class Name (localized)"="Application"}, "Method Info"={"Unique ID string"="834", "Data name"="XNode.Open", "Short name (localized)"="XNode.Open", "Long name (localized)"="XNode:Open"}, "Method Flags"={"IsDeprecated"=FALSE, "IsPrivate"=TRUE, "IsScripting"=FALSE, "IsNotInRun-Time"=TRUE}, "Divider"=FALSE}, {"Class Info"={"Unique ID string"="1", "Parent ID string"="", "Class Name (unlocalized)"="Application", "Class Name (localized)"="Application"}, "Method Info"={"Unique ID string"="835", "Data name"="Project.Load Default Project", "Short name (localized)"="Project.Load Default Project", "Long name (localized)"="Project:Load Default Project"}, "Method Flags"={"IsDeprecated"=FALSE, "IsPrivate"=TRUE, "IsScripting"=FALSE, "IsNotInRun-Time"=FALSE}, "Divider"=FALSE}, {"Class Info"={"Unique ID string"="1", "Parent ID string"="", "Class Name (unlocalized)"="Application", "Class Name (localized)"="Application"}, "Method Info"={"Unique ID string"="836", "Data name"="Get Shell Icon Of File", "Short name (localized)"="Get Shell Icon Of File", "Long name (localized)"="Get Shell Icon Of File"}, "Method Flags"={"IsDeprecated"=FALSE, "IsPrivate"=TRUE, "IsScripting"=FALSE, "IsNotInRun-Time"=FALSE}, "Divider"=FALSE}, {"Class Info"={"Unique ID string"="1", "Parent ID string"="", "Class Name (unlocalized)"="Application", "Class Name (localized)"="Application"}, "Method Info"={"Unique ID string"="837", "Data name"="Project.Get Icon Of Type", "Short name (localized)"="Project.Get Icon Of Type", "Long name (localized)"="Project:Get Icon Of Type"}, "Method Flags"={"IsDeprecated"=FALSE, "IsPrivate"=TRUE, "IsScripting"=FALSE, "IsNotInRun-Time"=FALSE}, "Divider"=FALSE}, {"Class Info"={"Unique ID string"="1", "Parent ID string"="", "Class Name (unlocalized)"="Application", "Class Name (localized)"="Application"}, "Method Info"={"Unique ID string"="839", "Data name"="UI.Invoke Prefs Dlg", "Short name (localized)"="UI.Invoke Prefs Dlg", "Long name (localized)"="User Interaction:Invoke Preferences Dialog"}, "Method Flags"={"IsDeprecated"=FALSE, "IsPrivate"=TRUE, "IsScripting"=FALSE, "IsNotInRun-Time"=FALSE}, "Divider"=FALSE}, {"Class Info"={"Unique ID string"="1", "Parent ID string"="", "Class Name (unlocalized)"="Application", "Class Name (localized)"="Application"}, "Method Info"={"Unique ID string"="83a", "Data name"="License.Get Licensed Version", "Short name (localized)"="License.Get Licensed Version", "Long name (localized)"="License:Get Licensed Version"}, "Method Flags"={"IsDeprecated"=FALSE, "IsPrivate"=TRUE, "IsScripting"=FALSE, "IsNotInRun-Time"=FALSE}, "Divider"=FALSE}, {"Class Info"={"Unique ID string"="1", "Parent ID string"="", "Class Name (unlocalized)"="Application", "Class Name (localized)"="Application"}, "Method Info"={"Unique ID string"="83c", "Data name"="Config.Set Settings", "Short name (localized)"="Config.Set Settings", "Long name (localized)"="Configuration:Set Settings"}, "Method Flags"={"IsDeprecated"=FALSE, "IsPrivate"=TRUE, "IsScripting"=FALSE, "IsNotInRun-Time"=FALSE}, "Divider"=FALSE}, {"Class Info"={"Unique ID string"="1", "Parent ID string"="", "Class Name (unlocalized)"="Application", "Class Name (localized)"="Application"}, "Method Info"={"Unique ID string"="83d", "Data name"="Config.Get Target App's Settings", "Short name (localized)"="Config.Get Target App's Settings", "Long name (localized)"="Configuration:Get Target App's Settings"}, "Method Flags"={"IsDeprecated"=FALSE, "IsPrivate"=TRUE, "IsScripting"=FALSE, "IsNotInRun-Time"=FALSE}, "Divider"=FALSE}, {"Class Info"={"Unique ID string"="1", "Parent ID string"="", "Class Name (unlocalized)"="Application", "Class Name (localized)"="Application"}, "Method Info"={"Unique ID string"="83e", "Data name"="Config.Set Target App's Settings", "Short name (localized)"="Config.Set Target App's Settings", "Long name (localized)"="Configuration:Set Target App's Settings"}, "Method Flags"={"IsDeprecated"=FALSE, "IsPrivate"=TRUE, "IsScripting"=FALSE, "IsNotInRun-Time"=FALSE}, "Divider"=FALSE}, {"Class Info"={"Unique ID string"="1", "Parent ID string"="", "Class Name (unlocalized)"="Application", "Class Name (localized)"="Application"}, "Method Info"={"Unique ID string"="83f", "Data name"="Global Data.Set", "Short name (localized)"="Global Data.Set", "Long name (localized)"="Global Data:Set"}, "Method Flags"={"IsDeprecated"=FALSE, "IsPrivate"=TRUE, "IsScripting"=FALSE, "IsNotInRun-Time"=FALSE}, "Divider"=FALSE}, {"Class Info"={"Unique ID string"="1", "Parent ID string"="", "Class Name (unlocalized)"="Application", "Class Name (localized)"="Application"}, "Method Info"={"Unique ID string"="840", "Data name"="Global Data.Get", "Short name (localized)"="Global Data.Get", "Long name (localized)"="Global Data:Get"}, "Method Flags"={"IsDeprecated"=FALSE, "IsPrivate"=TRUE, "IsScripting"=FALSE, "IsNotInRun-Time"=FALSE}, "Divider"=FALSE}, {"Class Info"={"Unique ID string"="1", "Parent ID string"="", "Class Name (unlocalized)"="Application", "Class Name (localized)"="Application"}, "Method Info"={"Unique ID string"="841", "Data name"="Global Data.Free", "Short name (localized)"="Global Data.Free", "Long name (localized)"="Global Data:Free"}, "Method Flags"={"IsDeprecated"=FALSE, "IsPrivate"=TRUE, "IsScripting"=FALSE, "IsNotInRun-Time"=FALSE}, "Divider"=FALSE}, {"Class Info"={"Unique ID string"="1", "Parent ID string"="", "Class Name (unlocalized)"="Application", "Class Name (localized)"="Application"}, "Method Info"={"Unique ID string"="843", "Data name"="Linker.Write Info To File", "Short name (localized)"="Linker.Write Info To File", "Long name (localized)"="Linker:Write Info To File"}, "Method Flags"={"IsDeprecated"=FALSE, "IsPrivate"=TRUE, "IsScripting"=FALSE, "IsNotInRun-Time"=TRUE}, "Divider"=FALSE}, {"Class Info"={"Unique ID string"="1", "Parent ID string"="", "Class Name (unlocalized)"="Application", "Class Name (localized)"="Application"}, "Method Info"={"Unique ID string"="844", "Data name"="DbgConn.OpenDbgConn", "Short name (localized)"="DbgConn.OpenDbgConn", "Long name (localized)"="Debug Connection:Open Debug Connection"}, "Method Flags"={"IsDeprecated"=FALSE, "IsPrivate"=FALSE, "IsScripting"=FALSE, "IsNotInRun-Time"=TRUE}, "Divider"=FALSE}, {"Class Info"={"Unique ID string"="1", "Parent ID string"="", "Class Name (unlocalized)"="Application", "Class Name (localized)"="Application"}, "Method Info"={"Unique ID string"="845", "Data name"="DbgConn.CloseDbgConn", "Short name (localized)"="DbgConn.CloseDbgConn", "Long name (localized)"="Debug Connection:Close Debug Connection"}, "Method Flags"={"IsDeprecated"=FALSE, "IsPrivate"=FALSE, "IsScripting"=FALSE, "IsNotInRun-Time"=TRUE}, "Divider"=FALSE}, {"Class Info"={"Unique ID string"="1", "Parent ID string"="", "Class Name (unlocalized)"="Application", "Class Name (localized)"="Application"}, "Method Info"={"Unique ID string"="846", "Data name"="DbgConn.ListApps", "Short name (localized)"="DbgConn.ListApps", "Long name (localized)"="Debug Connection:List Applications or Shared Libraries"}, "Method Flags"={"IsDeprecated"=FALSE, "IsPrivate"=FALSE, "IsScripting"=FALSE, "IsNotInRun-Time"=TRUE}, "Divider"=FALSE}, {"Class Info"={"Unique ID string"="1", "Parent ID string"="", "Class Name (unlocalized)"="Application", 
